vi "AddRoom.vi"(8 "error in (no error)":errorcluster, 10 "Room*":refnum<data-value>, 11 "Maze in":refnum<class "Maze.lvclass">) -> (0 "error out":errorcluster, 3 "Maze out":refnum<class "Maze.lvclass">)   [LabVIEW 2016, in "Maze.lvclass"]
uses:
  Maze.lvclass
  Room/Room.lvclass
  Maze.lvclass/Maze.ctl
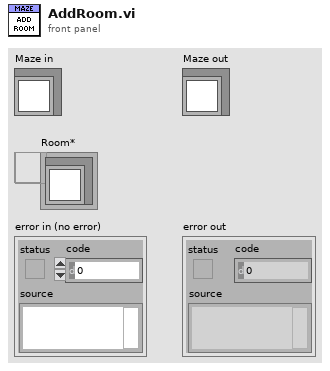
[diagram p1: front panel]
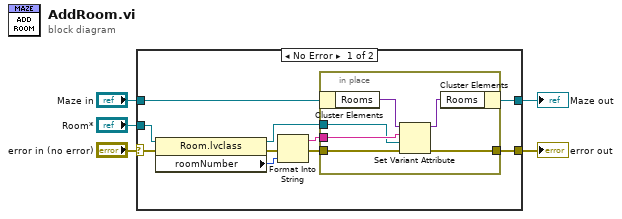
[diagram p0: block diagram]
diagram:
  n1 = case shown="No Error" "error in (no error)" {
    selector: "error in (no error)" -> [w10 w23]
    tunnel: [w6 w23] -> w4
    tunnel: [w14 w22] -> w2
    tunnel: "Maze in" -> [w15 w22]
    tunnel: "Room*" -> [w11 _]
    frame No Error {
      n2 = property class="Room.lvclass"(reference=w11, error in=w10) -> (reference out=w9:refnum<data-value>, error out=w8:errorcluster, "roomNumber"=w13:i32)
      n3 = Format Into String(error in=w8, w13) -> (resulting string=w12:string, error out=w7:errorcluster)  [unwired: 2 in]
      n4 = in-place {
        in-place-border: w12 -> [w19]
        in-place-border: w9 -> [w18]
        in-place-border: w7 -> [w17]
        in-place-border: [w16] -> w6
        n5 = in-place-cluster #1(w15) -> ("Rooms"=w21:variant)
        n6 = Set Variant Attribute(Variant=w21, name=w19, value=w18, error in=w17) -> (Variant out=w20:variant, error out=w16:errorcluster)  [unwired: 1 out]
        n7 = in-place-cluster #1("Rooms"=w20) -> (w14:refnum<class "Maze.lvclass">)
      }
    }
    frame Error {
    }
  }
  "error out" <- w4
  "Maze out" <- w2
